vi "Open Instrument.vi"(8 "error in (no error)":errorcluster, 11 "instrument.PPMS":refnum<class "instrument.PPMS.lvclass">) -> (0 "error out":errorcluster, 3 "instrument.PPMS out":refnum<class "instrument.PPMS.lvclass">)   [LabVIEW 2019, in "instrument.PPMS.lvclass"]
uses:
  instrument.PPMS.lvclass
  C:/Program Files (x86)/National Instruments/LabVIEW 2019/user.lib/LevyLab/Levylab Instruments/SMOs/Instrument/Instrument.lvclass
  <userlib>/LevyLab/Levylab Instruments/SMOs/Instrument/Instrument.lvclass/Instrument.ctl
  instrument.PPMS.lvclass/instrument.PPMS.ctl
  <userlib>/LevyLab/Levylab Instruments/SMOs/Instrument/Instrument.lvclass
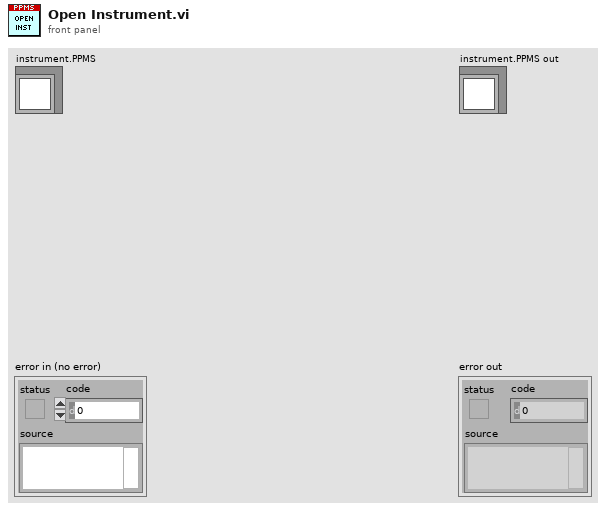
[diagram p1: front panel]
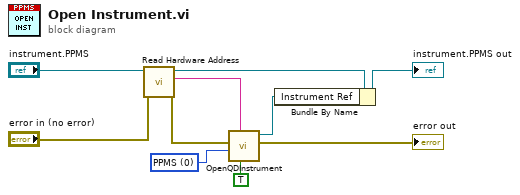
[diagram p0: block diagram]
diagram:
  w9 = 0 items=["PPMS", "VersaLab", "DynaCool", "SVSM"] ("Instrument\nType")
  n1 = call <userlib>:"Read Hardware Address.vi"("error in (no error)"="error in (no error)", "Instrument in"="instrument.PPMS") -> ("error out"=w1:errorcluster, "Address"=w7:string, "Instrument out"=w5:refnum<class "instrument.PPMS.lvclass">)  [unwired: 7 in]
  n2 = call "OpenQDInstrument.vi"("Remote"=TRUE, "IP Address"=w7, "Instrument Type"=w9, "error in (no error)"=w1) -> ("error out"=→"error out":errorcluster, "Instrument Ref"=w3:refnum<k24>)  [unwired: 4 in]
  n3 = Bundle By Name(cluster=w5, "Instrument Ref"=w3) -> (→"instrument.PPMS out":refnum<class "instrument.PPMS.lvclass">)
